vi "entry type constant.vi"() -> (0 "map":T1)   [LabVIEW 2024, in "controls manager.lvlib"]
uses:
  controls manager.lvlib
  collection type.ctl
  entry type.ctl
  control.ctl
  controls plan.ctl
  key value pair.ctl
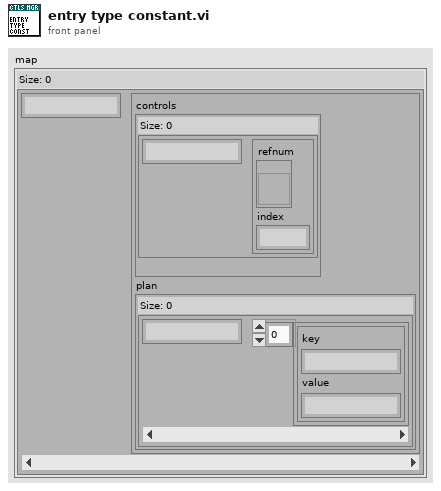
[diagram p1: front panel]
types:
  T1 = typedef "controls manager.lvlib/collection type.ctl" = map{string, T2}
  T2 = typedef "controls manager.lvlib/entry type.ctl" = cluster{"controls":map{string, T3}, "plan":T4}
  T3 = typedef "controls manager.lvlib/control.ctl" = cluster{"refnum":refnum<vi>, "index":i32}
  T4 = typedef "controls manager.lvlib/controls plan.ctl" = map{string, T5[]}
  T5 = typedef "controls manager.lvlib/key value pair.ctl" = cluster{"key":string, "value":string}
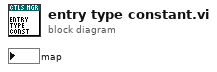
[diagram p0: block diagram]
diagram:
